vi "Select Active Channels.vi"(8 "error in (no error)":errorcluster, 10 "Active Channel(s)":T1[](array[typedef]), 11 "PXIe5105 in":refnum<class "PXIe5105.lvclass">) -> (0 "error out":errorcluster, 3 "PXIe5105 out":refnum<class "PXIe5105.lvclass">)   [LabVIEW 2018, in "PXIe5105.lvlib" / "PXIe5105.lvclass"]
doc: "This Override method is used to set active channels for the Oscope. Use the 'Active Channel(s)' control to select channel(s)."
uses:
  PXIe5105.lvclass
  PPLs/Oscilloscope/Parent/Oscilloscope.lvlibp/Custom Controls/Analog Channels.ctl
  PXIe5105.lvclass/PXIe5105.ctl
  PPLs/Oscilloscope/Parent/Oscilloscope.lvlibp
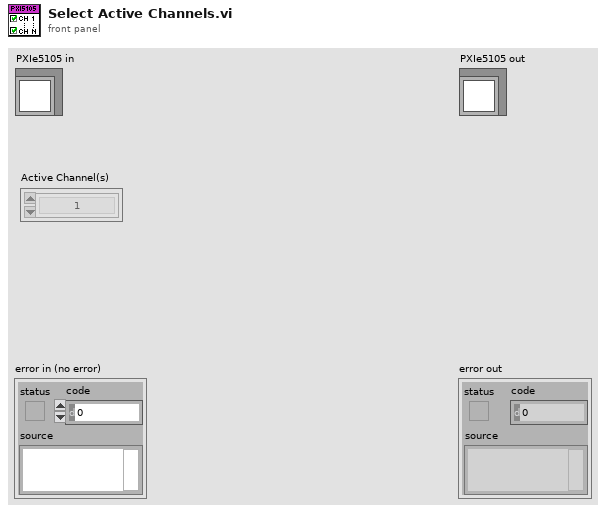
[diagram p1: front panel]
types:
  T1 = typedef "Oscilloscope.lvlibp/Analog Channels.ctl" = enum16{"1", "2", "3", "4", "5", "6", "7", "8", "9", "10", "11", "12", "13", "14", "15", "16"}
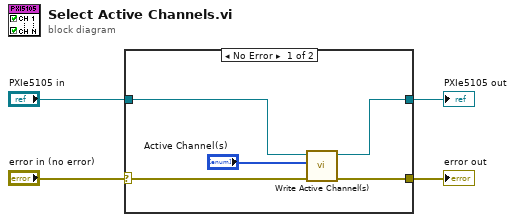
[diagram p0: block diagram]
diagram:
  n1 = case shown="No Error" "error in (no error)" {
    selector: "error in (no error)" -> [w7 w11]
    tunnel: [w6 w11] -> w3
    tunnel: "PXIe5105 in" -> [w9 w10]
    tunnel: [w5 w10] -> w1
    frame No Error {
      n2 = call "Write Active Channel(s).vi"("error in (no error)"=w7, "Active Channel(s)"="Active Channel(s)", "PXIe5105 in"=w9) -> ("error out"=w6:errorcluster, "PXIe5105 out"=w5:refnum<class "PXIe5105.lvclass">)  [unwired: 7 in]
    }
    frame Error {
    }
  }
  "error out" <- w3
  "PXIe5105 out" <- w1
